vi "sequentialdeviation.vi"() -> ()   [LabVIEW 2018]
panel:
  in  "C":dbl
  out "BIGGEST NUMBER":dbl
  in  "B":dbl
  in  "A":dbl
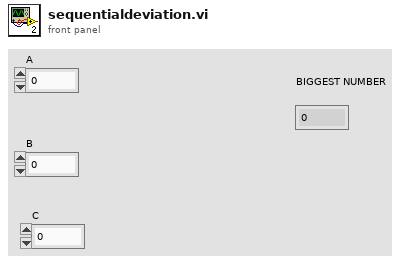
[diagram p1: front panel]
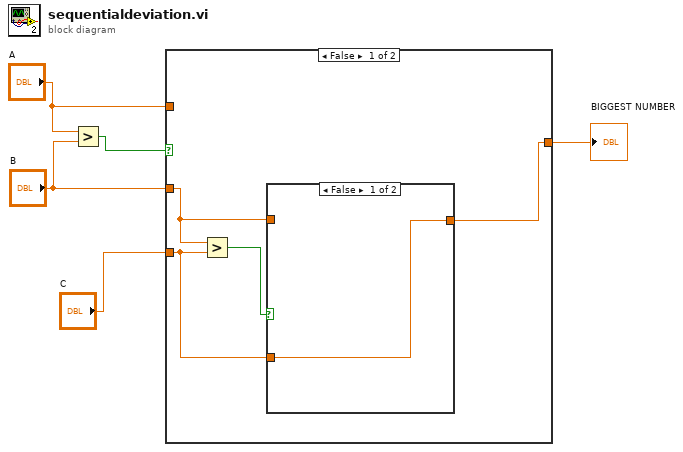
[diagram p0: block diagram]
diagram:
  n1 = Greater?(x="A", y="B") -> (0:w3:bool)
  n2 = case shown="False" w3 {
    tunnel: "A" -> [_ w12]
    tunnel: [w6 w12] -> w4
    tunnel: "B" -> [w8 _]
    tunnel: "C" -> [w9 _]
    frame False {
      n3 = Greater?(x=w8, y=w9) -> (0:w7:bool)
      n4 = case shown="False" w7 {
        tunnel: w9 -> [w10 _]
        tunnel: w8 -> [_ w11]
        tunnel: [w10 w11] -> w6
        frame False {
        }
        frame True {
        }
      }
    }
    frame True {
    }
  }
  "BIGGEST NUMBER" <- w4
